vi "Config D-A Output Time.vi"(0 "VISA resource name":refnum<visa-resource-name>, 5 "Hour (1)":u32=1 max=10000, 7 "Minute (0)":u32 max=59 step=1, 9 "Second (0)":u32 max=59 step=1, 11 "error in (no error)":errorcluster) -> (4 "VISA resource name out":refnum<visa-resource-name>, 15 "error out":errorcluster)   [LabVIEW 2010, in "Yokogawa WT200 Series.lvlib"]
doc: "This VI sends the preset integration time for D/A output of integrated values to the WT200 Series.\n\nNote : It needs /D4, /D12, /CMP option."
uses:
  G:/Engineering/Retail/LabV/instr.lib/Yokogawa WT200 Series/Yokogawa WT200 Series.lvlib
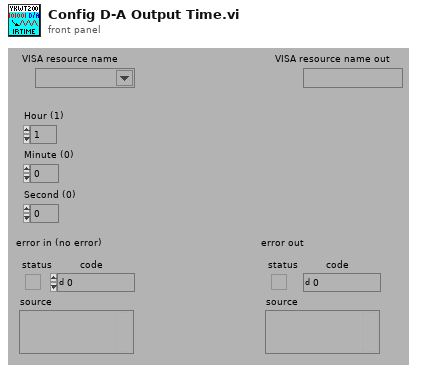
[diagram p1: front panel]
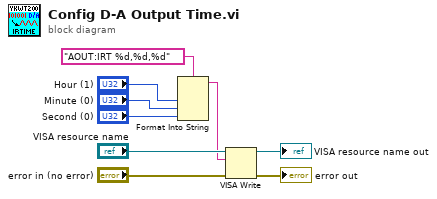
[diagram p0: block diagram]
diagram:
  n1 = Format Into String(format string="AOUT:IRT %d,%d,%d", "Hour (1)", "Minute (0)", "Second (0)") -> (resulting string=w5:string)  [unwired: 2 in, 1 out]
  n2 = VISA Write(VISA resource name="VISA resource name", write buffer=w5, error in (no error)="error in (no error)") -> (VISA resource name out=→"VISA resource name out":refnum<visa-resource-name>, error out=→"error out":errorcluster)  [unwired: 1 out]
